vi "Get Connected Caves.vi"(10 "Cave":T1, 11 "All Caves":T1[](array[typedef])) -> (3 "Connected Caves":T1[](array[typedef]))   [LabVIEW 2019, in "Day 12.lvlib"]
uses:
  Day 12.lvlib
  Controls/Cave.ctl
  Controls/Cave Type.ctl
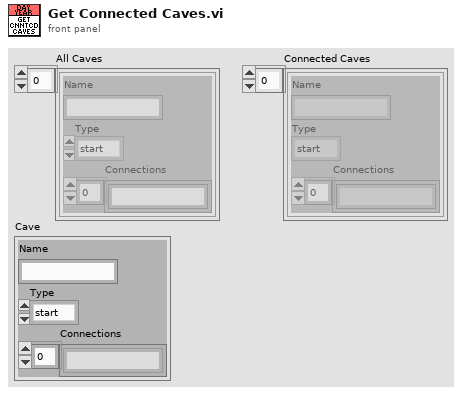
[diagram p1: front panel]
types:
  T1 = typedef "Day 12.lvlib/Cave.ctl" = cluster{"Name":string, "Type":T2, "Connections":string[]}
  T2 = typedef "Day 12.lvlib/Cave Type.ctl" = enum16{"start", "end", "small", "big"}
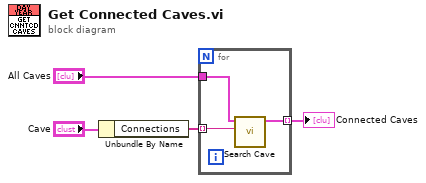
[diagram p0: block diagram]
diagram:
  n1 = Unbundle By Name("Cave") -> ("Connections"=w1:string[])
  n2 = for {
    tunnel: w1 -> [w6] mode=indexing
    tunnel: "All Caves" -> [w7]
    tunnel: [w5] -> w3 mode=indexing
    n3 = call "Search Cave.vi"("Cave Name"=w6, "Caves"=w7) -> ("Cave"=w5:T1)  [unwired: 7 in, 2 out]
  }
  "Connected Caves" <- w3
